vi "Read Data Strings.vi"(8 "error in (no error)":errorcluster, 11 "Run System Exec in":refnum<class "Run System Exec.lvclass">) -> (0 "error out":errorcluster, 1 "standard input":string, 2 "command line":string, 3 "Run System Exec out":refnum<class "Run System Exec.lvclass">)   [LabVIEW 2019, in "ProjectBuilder.lvlib" / "Run System Exec.lvclass"]
doc: "Read private data."
uses:
  Run System Exec.lvclass
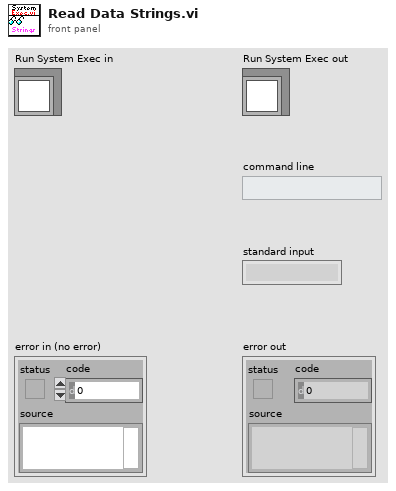
[diagram p1: front panel]
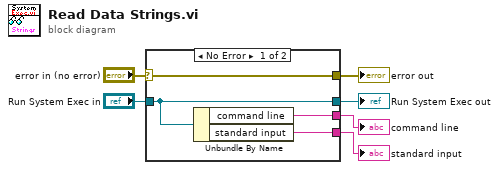
[diagram p0: block diagram]
diagram:
  n1 = case shown="No Error" "error in (no error)" {
    selector: "error in (no error)" -> [w10 w11]
    tunnel: [w10 w11] -> w5
    tunnel: [w9 w12] -> w3
    tunnel: "Run System Exec in" -> [w9 w12]
    tunnel: [w8 _] -> w2
    tunnel: [w7 _] -> w1
    frame No Error {
      n2 = Unbundle By Name(w9) -> ("command line"=w8:string, "standard input"=w7:string)
    }
    frame Error {
    }
  }
  "error out" <- w5
  "Run System Exec out" <- w3
  "command line" <- w2
  "standard input" <- w1
